vi "Read Multiple Channels.vi"(8 "error in (no error)":errorcluster, 10 "Channel Array":refnum<k21>[](array[refnum]), 11 "Timing":T1 {"Sampling Mode" items=["Finite Samples"=10178, "Continuous Samples"=10123, "Hardware Timed Single Point"=12522]; "Sampling Rate (Hz)" format="%0.2f"}) -> (0 "error out":errorcluster, 3 "data":waveform(dbl)[][](array[waveform]))   [LabVIEW 2017]
uses:
  Controls/Timing Controls.ctl
  <vilib>/DAQmx/read.llb/DAQmx Read (Analog 1D Wfm NChan NSamp).vi
  <vilib>/DAQmx/miscellaneous.llb/DAQmx Fill In Error Info.vi
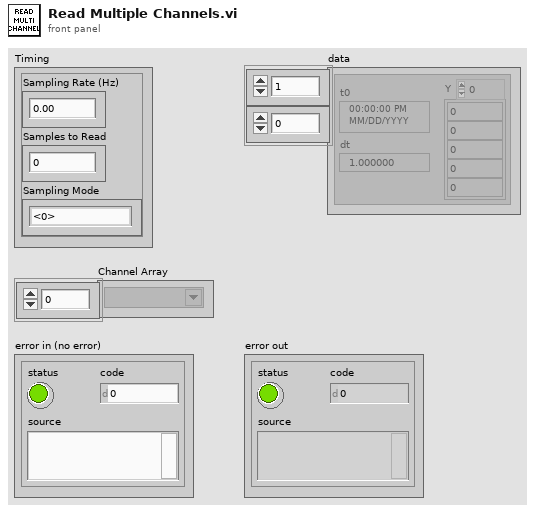
[diagram p1: front panel]
types:
  T1 = typedef "Timing Controls.ctl" = cluster{"Sampling Rate (Hz)":dbl, "Samples to Read":i32, "Sampling Mode":i32}
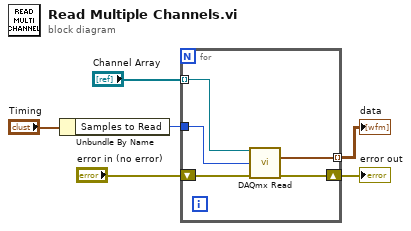
[diagram p0: block diagram]
diagram:
  n1 = Unbundle By Name("Timing") -> ("Samples to Read"=w3:i32)
  n2 = for {
    tunnel: [w10] -> w4 mode=indexing
    tunnel: w3 -> [w8]
    shift-right: [w9] -> w5
    shift-left: "error in (no error)" -> [w11]
    tunnel: "Channel Array" -> [w7] mode=indexing
    n3 = call-poly <vilib>:"DAQmx Read.vi"("task/channels in"=w7, "number of samples per channel"=w8, "error in"=w11) -> ("data"=w10:waveform(dbl)[], "error out"=w9:errorcluster)  [unwired: 10 in, 1 out]
  }
  "error out" <- w5
  "data" <- w4
